vi "Run.vi"(9 "Team In":refnum<class "Team.lvclass">, 11 "MySquare in":refnum<class "MySquare.lvclass">) -> (1 "Team":refnum<class "Team.lvclass">, 2 "Run Result":T1, 3 "MySquare out":refnum<class "MySquare.lvclass">)   [LabVIEW 2020, in "SquareTeam.lvlib" / "MySquare.lvclass"]
doc: "This VI is called on every active square each turn of the game for the square to decide what action to take."
uses:
  MySquare.lvclass
  SquareBattle/Run Result.ctl
  SquareBattle/Square/Square.lvclass
  SquareBattle/Action.ctl
  SquareBattle/Direction.ctl
  SquareBattle/Team/Team.lvclass
  MyTeam/MyTeam.lvclass
  C:/dev/sol-squarebattle/SquareBattle/Team/Team.lvclass
  SquareBattle/SquareBattle.lvlib
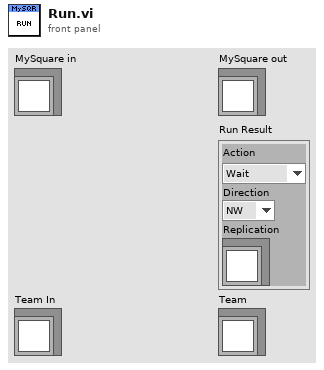
[diagram p1: front panel]
types:
  T1 = typedef "SquareBattle.lvlib/Run Result.ctl" = cluster{"Action":T2, "Direction":T3, "Replication":refnum<class "Square.lvclass">}
  T2 = typedef "SquareBattle.lvlib/Action.ctl" = enum16{"Wait", "Move", "Attack", "Replicate"}
  T3 = typedef "SquareBattle.lvlib/Direction.ctl" = enum16{"NW", "N", "NE", "E", "SE", "S", "SW", "W"}
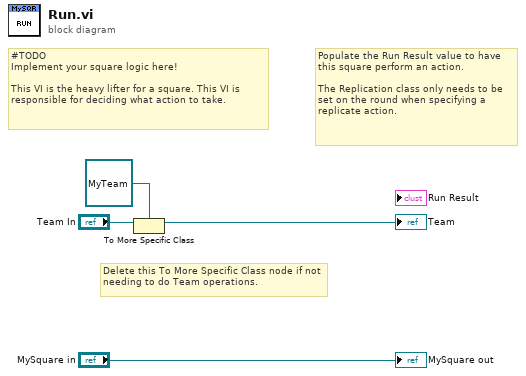
[diagram p0: block diagram]
diagram:
  # "Populate the Run Result value to have this square perform an action.\n\nThe Replication class only needs to be set on the round when specifying a replicate action."
  # "#TODO\nImplement your square logic here!\n\nThis VI is the heavy lifter for a square. This VI is responsible for deciding what action to take."
  # "Delete this To More Specific Class node if not needing to do Team operations."
  n1 = To More Specific Class(target class=refnum<class "MyTeam.lvclass"> refnum ("SquareTeam.lvlib:MyTeam.lvclass"), reference="Team In") -> (specific class reference=→"Team":refnum<class "MyTeam.lvclass">)  [unwired: 1 in, 1 out]
  "MySquare out" <- "MySquare in"
